vi "Log Data.vi"(0 "Test Inputs":T2 {"Nominal Output Voltage in V" format="%#.5g"; "Input Voltage in V" format="%#.5g"}, 5 "Test Results":T1 {"Load Regulation in mV/mA" format="%#.5g"; "Measured Input Voltage in V" format="%#.5g"; "Measured Input Current in A" format="%#.5g"; "Measured Load Current in A" format="%#.5g"; "Load Regulation in Percentage" format="%#.3g"; "Measured Output Voltage in V" format="%#.5g"}, 7 "DataLogger File Path":path, 11 "error in (no error)":errorcluster) -> (15 "error out":errorcluster)   [LabVIEW 2020, in "LDO Load Regulation.lvlib"]
uses:
  LDO Load Regulation.lvlib
  Typedefs/Test Inputs.ctl
  Typedefs/Advance Settings.ctl
  Typedefs/Adv Setup.ctl
  Reusables/Instrument APIs/Load Output Function.ctl
  Typedefs/Adv StimulusMeasure.ctl
  Typedefs/Test Results.ctl
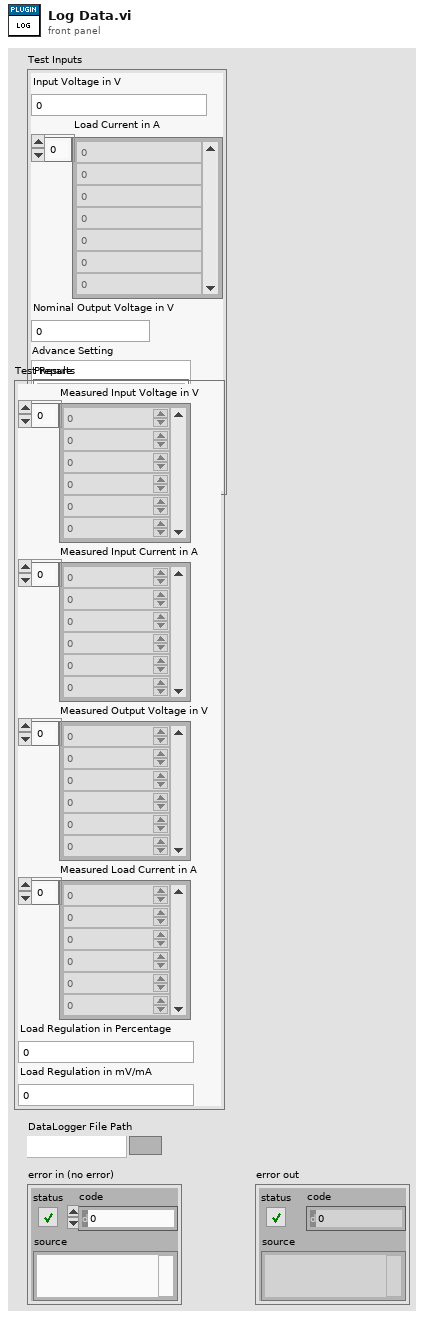
[diagram p1: front panel]
types:
  T1 = typedef "LDO Load Regulation.lvlib/Test Results.ctl" = cluster{"Measured Input Voltage in V":dbl[], "Measured Input Current in A":dbl[], "Measured Output Voltage in V":dbl[], "Measured Load Current in A":dbl[], "Load Regulation in Percentage":dbl, "Load Regulation in mV/mA":dbl}
  T2 = typedef "LDO Load Regulation.lvlib/Test Inputs.ctl" = cluster{"Input Voltage in V":dbl, "Load Current in A":dbl[], "Nominal Output Voltage in V":dbl, "Advance Setting":T3}
  T3 = typedef "LDO Load Regulation.lvlib/Advance Settings.ctl" = cluster{"Prepare":T4, "Stimulus And Measure":T6}
  T4 = typedef "LDO Load Regulation.lvlib/Adv Setup.ctl" = cluster{"Load SMU Output Function":T5}
  T5 = typedef "Load Output Function.ctl" = enum16{"VoltageSource", "CurrentSource"}
  T6 = typedef "LDO Load Regulation.lvlib/Adv StimulusMeasure.ctl" = cluster{"Loop Delay in milliSecond":u32}
  T7 = enum16{"open", "replace", "create", "open or create", "replace or create", "replace or create with confirmation"}
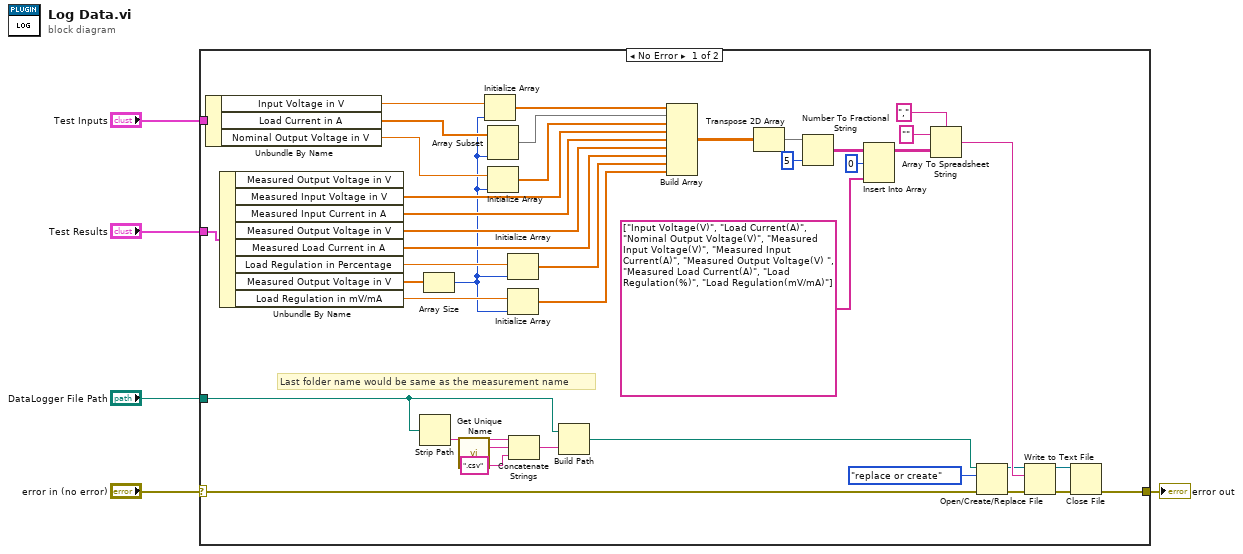
[diagram p0: block diagram]
diagram:
  n1 = case shown="No Error" "error in (no error)" {
    selector: "error in (no error)" -> [w20 w47]
    tunnel: [w28 w47] -> w4
    tunnel: "Test Inputs" -> [w46 _]
    tunnel: "Test Results" -> [w45 _]
    tunnel: "DataLogger File Path" -> [w11 _]
    frame No Error {
      # "Last folder name would be same as the measurement name"
      n2 = Unbundle By Name(w46) -> ("Input Voltage in V"=w33:dbl, "Load Current in A"=w23:dbl[], "Nominal Output Voltage in V"=w35:dbl)
      n3 = Unbundle By Name(w45) -> ("Measured Input Voltage in V"=w40:dbl[], "Measured Input Current in A"=w41:dbl[], "Measured Output Voltage in V"=w42:dbl[], "Measured Load Current in A"=w43:dbl[], "Load Regulation in Percentage"=w31:dbl, "Measured Output Voltage in V"=w29:dbl[], "Load Regulation in mV/mA"=w8:dbl)  [unwired: 1 out]
      n4 = Strip Path(path=w11) -> (name=w13:string)  [unwired: 1 out]
      n5 = Array Size(array=w29) -> (size(s)=w7:i32)
      n6 = call "Get Unique Name.vi"() -> ("Unique String"=w14:string)  [unwired: 14 in, 1 out]
      n7 = Initialize Array(w33, w7) -> (w32:dbl[])
      n8 = Array Subset(array=w23, length=w7) -> (w22:dbl[])  [unwired: 1 in]
      n9 = Initialize Array(w35, w7) -> (w34:dbl[])
      n10 = Initialize Array(w31, w7) -> (w30:dbl[])
      n11 = Initialize Array(w8, w7) -> (w6:dbl[])
      n12 = Concatenate Strings(w13, w14, ".csv" ("format string")) -> (w10:string)
      n13 = Build Path(base path=w11, name or relative path=w10) -> (appended path=w9:path)
      n14 = Build Array(w32, w22, w34, w40, w41, w42, w43, w30, w6) -> (w39:dbl[][])
      n15 = Transpose 2D Array(2D array=w39) -> (transposed array=w44:dbl[][])
      n16 = Number To Fractional String(number=w44, precision (6)=i16 5) -> (F-format string=w36:string[][])  [unwired: 2 in]
      n17 = Insert Into Array(array=w36, index (row)=0, new element=string[] ["Input Voltage(V)", "Load Current(A)", "Nominal Output Voltage(V)", "Measured Input Voltage(V)", "Measured Input Current(A)", "Measured Output Voltage(V) ", "Measured Load Current(A)", "Load Regulation(%)", "Load Regulation(mV/mA)"] ("new element/subarray")) -> (w25:string[][])  [unwired: 1 in]
      n18 = Array To Spreadsheet String(delimiter (Tab)=",", array=w25, 3:"" ("format string")) -> (spreadsheet string=w24:string)
      n19 = Open/Create/Replace File(file path (use dialog)=w9, error in=w20, operation (0:open)=T7."replace or create") -> (refnum out=w17:refnum<file>, error out=w19:errorcluster)  [unwired: 3 in, 1 out]
      n20 = Write to Text File(file (use dialog)=w17, text=w24, error in=w19) -> (refnum out=w16:refnum<file>, error out=w18:errorcluster)  [unwired: 1 in, 1 out]
      n21 = Close File(refnum=w16, error in=w18) -> (error out=w28:errorcluster)  [unwired: 1 out]
    }
    frame Error {
    }
  }
  "error out" <- w4
